vi "ProceListAction2.vi"(9 "Btn_AutoRun":refnum<vi>, 11 "AutoRunFlg":refnum<vi>) -> (0 "error out":errorcluster, 2 "pause":bool)   [LabVIEW 2019]
uses:
  Ctrl/MainPage UI Ref_VirbVision.ctl
  Function/Main UI/Glb/Main_UI Gb.vi
  LLB/Message/MsgShowAndLog.lvlib
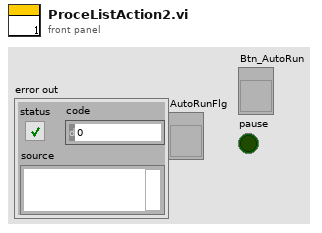
[diagram p1: front panel]
types:
  T1 = typedef "MainPage UI Ref_VirbVision.ctl" = cluster{"ProcessList":refnum<vi>, "Result Arr":refnum<vi>, "StopReceiveCmd":refnum<vi>}
  T2 = enum16{"Initial", "Write", "Read", "Save", "Load", "WrteAll"}
  T3 = enum16{"initial", "write", "add", "delete", "Load", "Save", "Read", "ReadProjectName"}
  T4 = cluster{"ProjectName":string, "Parameter":string[][]}[]
  T5 = cluster{"ProjectName":string, "Parameter":string[][]}
  T6 = cluster{"ROI":string, "Numbers":i32, "Data":string[][]}[]
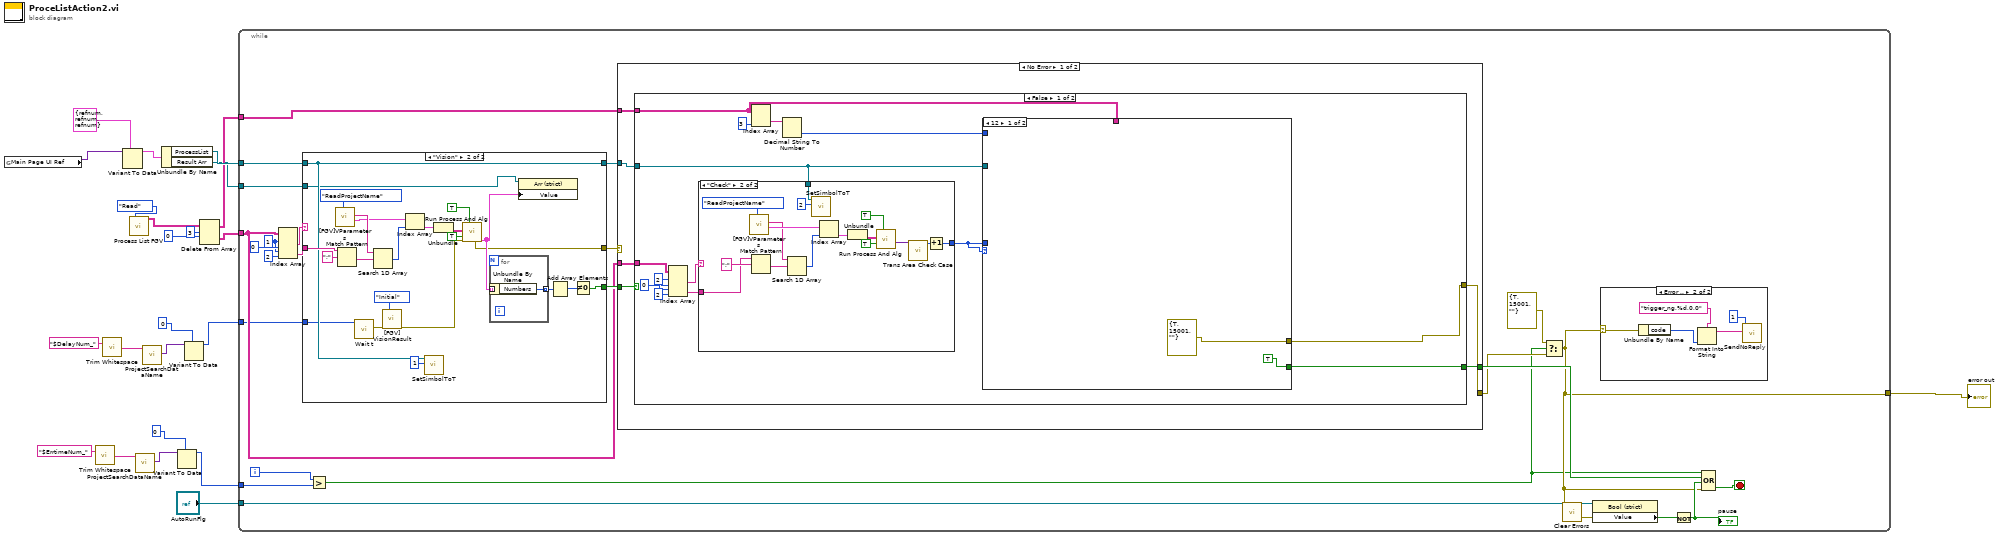
[diagram p0: block diagram]
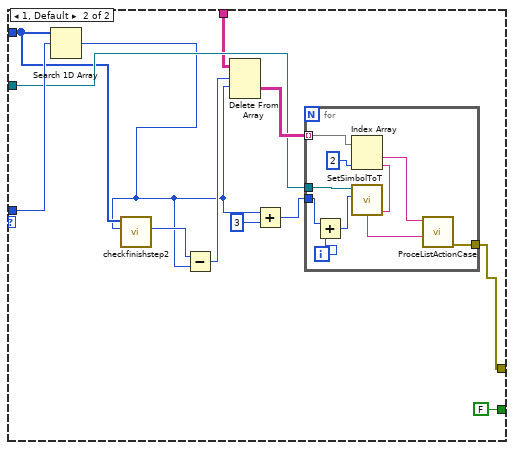
[diagram p2: hidden frame]
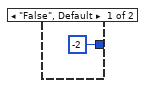
[diagram p3: hidden frame]
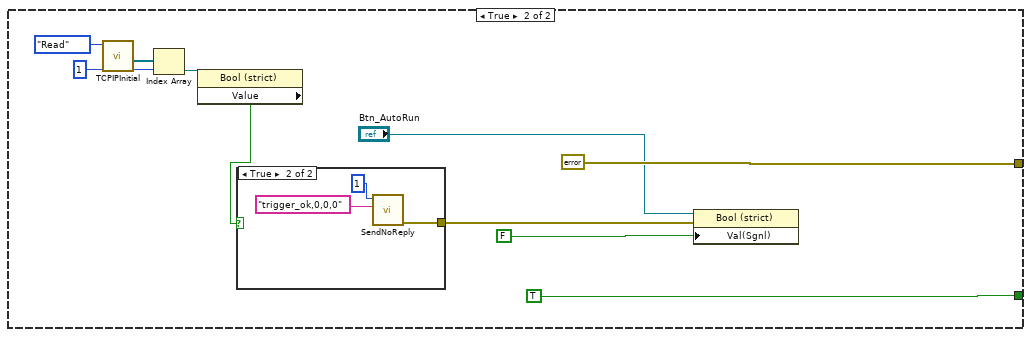
[diagram p4: hidden frame]
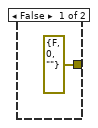
[diagram p5: hidden frame]
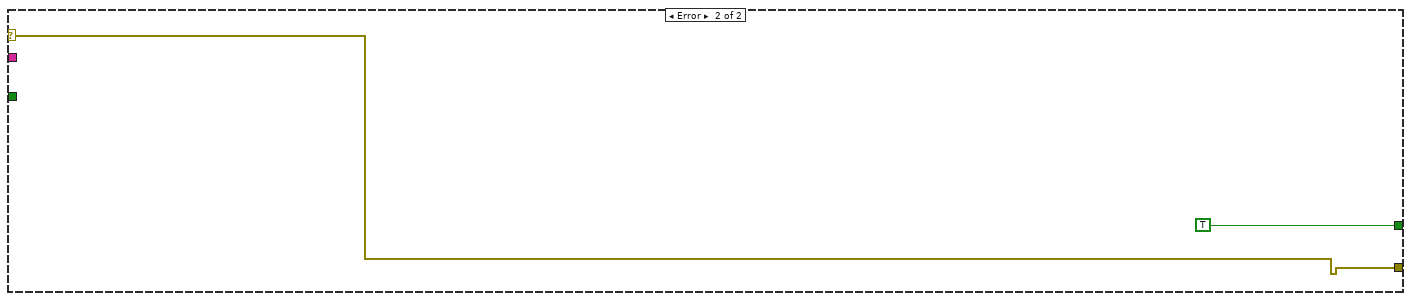
[diagram p6: hidden frame]
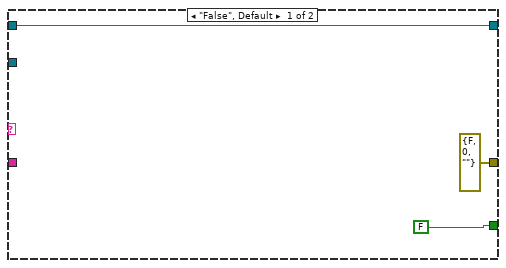
[diagram p7: hidden frame]
diagram:
  n1 = global read "Main_UI Gb.vi" "Main Page UI Ref"() -> (w2:variant)
  n2 = call <vilib>:"Trim Whitespace.vi"("string"="$ErrtimeNum_" ("element")) -> ("trimmed string"=w10:string)  [unwired: 1 in]
  n3 = call <vilib>:"Trim Whitespace.vi"("string"="$DelayNum_" ("element")) -> ("trimmed string"=w9:string)  [unwired: 1 in]
  n4 = Variant To Data(type=T1 {"ProcessList"=refnum, "Result Arr"=refnum, "StopReceiveCmd"=refnum} ("Main Page UIRef"), Variant=w2) -> (data=w4:T1)  [unwired: 1 in, 1 out]
  n5 = call "Process List FGV.vi"("Action"=T2."Read") -> ("TableOut"=w19:string[][])  [unwired: 12 in, 2 out]
  n6 = call "ProjectSearchDataName.vi"("element"=w10) -> ("variant"=w13:variant)  [unwired: 7 in, 3 out]
  n7 = call "ProjectSearchDataName.vi"("element"=w9) -> ("variant"=w8:variant)  [unwired: 7 in, 3 out]
  n8 = Unbundle By Name(w4) -> ("ProcessList"=w22:refnum<vi>, "Result Arr"=w1:refnum<vi>)
  n9 = Variant To Data(type=0, Variant=w13) -> (data=w11:i32)  [unwired: 1 in, 1 out]
  n10 = Variant To Data(type=0, Variant=w8) -> (data=w5:i32)  [unwired: 1 in, 1 out]
  n11 = Delete From Array(array=w19, length=3, index (row)=0) -> (deleted portion=w16:string[][], array with subset deleted=w15:string[][])  [unwired: 1 in]
  n12 = while {
    tunnel: [w28] -> w21
    tunnel: w22 -> [w46]
    tunnel: "AutoRunFlg" -> [w44]
    tunnel: w16 -> [w33]
    tunnel: w15 -> [w32]
    tunnel: w11 -> [w30]
    tunnel: w5 -> [w25]
    tunnel: w1 -> [w24]
    i -> [w31]
    stop <- w48 stop-if-true
    w36 = 1 ("index (row)")
    n13 = Index Array(array=w33, index (row) #1=w36, index (col) #1=0 ("disabled index (col)"), index (row) #2=w36, index (col) #2=2 ("disabled index (col)")) -> (element #1=w37:string, element #2=w34:string)
    n14 = case shown="\"Vision\"" w37 {
      tunnel: w34 -> [_ w150]
      tunnel: [FALSE ("VisionOK") w138] -> w41
      tunnel: [w126 w131] -> w40
      tunnel: w46 -> [w126 w131]
      tunnel: [errorcluster {"status"=FALSE, "code"=0, "source"=""} ("error out") w132] -> w39
      tunnel: w25 -> [_ w129]
      tunnel: w24 -> [_ w128]
      frame "False", Default {
      }
      frame "Vision" {
        n15 = call "[FGV]VParameters.vi"("Enum"=T3."ReadProjectName") -> ("Data"=w144:T4, "ProjectName"=w147:string[])  [unwired: 7 in, 2 out]
        n16 = Match Pattern(string=w150, regular expression=";") -> (after substring=w146:string)  [unwired: 1 in, 3 out]
        n17 = call "Wait t.vi"("wait(ms)"=w129) -> ("error out"=w134:errorcluster)  [unwired: 10 in]
        n18 = Search 1D Array(1D array=w147, element=w146) -> (index of element=w145:i32)  [unwired: 1 in]
        n19 = call "[FGV] VisionResult.vi"("Action"=T2."Initial", "error in"=w134) -> ("error out"=w139:errorcluster)  [unwired: 11 in, 2 out]
        n20 = Index Array(array=w144, index=w145) -> (element=w143:T5)
        n21 = call "SetSimbolToT.vi"("index"=1, "ProcessList"=w131) -> ()  [unwired: 10 in]
        n22 = Unbundle(w143) -> ("Parameter"=w142:string[][])  [unwired: 1 out]
        n23 = call "Run Process And Alg.vi"("Process"=TRUE, "error in (no error)"=w139, "CheckDist"=TRUE, "ROIList"=w142) -> ("Result Arr"=w137:T6, "error out"=w132:errorcluster)  [unwired: 3 in, 3 out]
        n24 = for {
          tunnel: w137 -> [w152] mode=indexing
          tunnel: [w151] -> w136 mode=indexing
          n25 = Unbundle By Name(w152) -> ("Numbers"=w151:i32)
        }
        n26 = property class="Arr (strict)"(reference=w128, "Value"=w137) -> ()  [unwired: 1 in, 2 out]
        n27 = Add Array Elements(numeric array=w136) -> (sum=w135:i32)
        n28 = Not Equal To 0?(x=w135) -> (x != 0?=w138:bool)
      }
    }
    n29 = Greater?(x=w31, y=w30) -> (0:w27:bool)
    n30 = case shown="No Error" w39 {
      selector: w39 -> [_ w123]
      tunnel: w41 -> [w54 _]
      tunnel: [w53 w123] -> w29
      tunnel: [w52 TRUE] -> w47
      tunnel: w40 -> [w51 _]
      tunnel: w33 -> [w50 _]
      tunnel: w32 -> [w49 _]
      frame No Error {
        n31 = case shown="False" w54 {
          tunnel: [w57 errorcluster {"status"=FALSE, "code"=0, "source"="視覺結束"} ("error out")] -> w53
          tunnel: [w56 TRUE] -> w52
          tunnel: w51 -> [w55 _]
          tunnel: w50 -> [w68 _]
          tunnel: w49 -> [w60 _]
          frame False {
            w67 = 2 ("index (row)")
            n32 = Index Array(array=w68, index (row) #1=w67, index (col) #1=0 ("disabled index (col)"), index (row) #2=w67, index (col) #2=2 ("disabled index (col)")) -> (element #1=w63:string, element #2=w64:string)
            n33 = case shown="\"Check\"" w63 {
              tunnel: w64 -> [_ w98]
              tunnel: [-2 w95] -> w58
              tunnel: w55 -> [_ w93]
              frame "False", Default {
              }
              frame "Check" {
                n34 = call "[FGV]VParameters.vi"("Enum"=T3."ReadProjectName") -> ("Data"=w104:T4, "ProjectName"=w101:string[])  [unwired: 7 in, 2 out]
                n35 = Match Pattern(string=w98, regular expression=";") -> (after substring=w102:string)  [unwired: 1 in, 3 out]
                n36 = Search 1D Array(1D array=w101, element=w102) -> (index of element=w103:i32)  [unwired: 1 in]
                n37 = call "SetSimbolToT.vi"("index"=2, "ProcessList"=w93) -> ()  [unwired: 10 in]
                n38 = Index Array(array=w104, index=w103) -> (element=w105:T5)
                n39 = Unbundle(w105) -> ("Parameter"=w106:string[][])  [unwired: 1 out]
                n40 = call "Run Process And Alg.vi"("Process"=TRUE, "CheckDist"=TRUE, "ROIList"=w106) -> ("DetectOut"=w97:variant[])  [unwired: 4 in, 4 out]
                n41 = call "Trans Area Check Case.vi"("ResultIn"=w97) -> ("Case"=w96:i32)  [unwired: 10 in]
                n42 = Increment(x=w96) -> (x+1=w95:i32)
              }
            }
            n43 = Index Array(array=w60, index (col)=3 ("disabled index (col)")) -> (element=w61:string[])  [unwired: 1 in]
            n44 = Decimal String To Number(string=w61) -> (number=w59:i32[])  [unwired: 2 in, 1 out]
            n45 = case shown="12" w58 {
              tunnel: w58 -> [_ w82]
              tunnel: w55 -> [_ w78]
              tunnel: w60 -> [_ w77]
              tunnel: w59 -> [_ w76]
              tunnel: [errorcluster {"status"=TRUE, "code"=15001, "source"=""} ("t") w75] -> w57
              tunnel: [TRUE FALSE] -> w56
              frame 12 {
              }
              frame 1, Default {
                n46 = Search 1D Array(1D array=w76, element=w82) -> (index of element=w72:i32)  [unwired: 1 in]
                n47 = call "checkfinishstep2.vi"("Index"=w72, "StepNumber"=w76) -> ("Index"=w81:i32)  [unwired: 7 in, 2 out]
                n48 = Subtract(x=w81, y=w72) -> (x-y=w79:i32)
                n49 = Delete From Array(array=w77, length=w79, index (row)=w72) -> (deleted portion=w80:string[][])  [unwired: 1 in, 1 out]
                n50 = Add(x=w72, y=3) -> (x+y=w73:i32)
                n51 = for {
                  tunnel: [w91] -> w75
                  tunnel: w80 -> [w90] mode=indexing
                  tunnel: w78 -> [w86]
                  tunnel: w73 -> [w83]
                  i -> [w85]
                  n52 = Add(x=w83, y=w85) -> (x+y=w84:i32)
                  n53 = Index Array(array=w90, index #2=2 ("index")) -> (element #1=w89:string, element #2=w88:string)  [unwired: 1 in]
                  n54 = call "SetSimbolToT.vi"("index"=w84, "ProcessList"=w86) -> ()  [unwired: 10 in]
                  n55 = call "ProceListActionCase.vi"("DataIn"=w88, "TypeIn"=w89) -> ("error out"=w91:errorcluster)  [unwired: 9 in]
                }
              }
            }
          }
          frame True {
            n56 = call "TCPIPInitial.vi"("Enum"=enum16{"initial", "Read", "release"}."Read") -> ("Connect"=w112:refnum<vi>[])  [unwired: 7 in, 3 out]
            n57 = Index Array(array=w112, index=1) -> (element=w110:refnum<vi>)
            n58 = property class="Bool (strict)"(reference=w110) -> ("Value"=w109:bool)  [unwired: 1 in, 2 out]
            n59 = case shown="True" w109 {
              tunnel: [errorcluster {"status"=FALSE, "code"=0, "source"=""} ("error out") w120] -> w115
              frame False {
              }
              frame True {
                n60 = call "SendNoReply.vi"("DataIn"="trigger_ok,0,0,0", "index"=1) -> ("error out"=w120:errorcluster)  [unwired: 9 in]
              }
            }
            n61 = property class="Bool (strict)"(reference="Btn_AutoRun", error in=w115, "Val(Sgnl)"=FALSE ("Value")) -> ()  [unwired: 2 out]
          }
        }
      }
      frame Error {
      }
    }
    n62 = Select(t=errorcluster {"status"=TRUE, "code"=15001, "source"=""}, s=w27, f=w29) -> (s? t:f=w28:errorcluster)
    n63 = call <vilib>:"Clear Errors.vi"("error in (no error)"=w28) -> ("error out"=w43:errorcluster)  [unwired: 5 in, 1 out]
    n64 = property class="Bool (strict)"(reference=w44, error in=w43) -> ("Value"=w45:bool)  [unwired: 2 out]
    n65 = case shown="Error .." w28 {
      selector: w28 -> [_ w156]
      frame No Error {
      }
      frame Error {
        n66 = Unbundle By Name(w156) -> ("code"=w154:i32)
        n67 = Format Into String(format string="trigger_ng,%d,0,0" ("DataIn"), w154) -> (resulting string=w153:string)  [unwired: 2 in, 1 out]
        n68 = call "SendNoReply.vi"("DataIn"=w153, "index"=1) -> ()  [unwired: 9 in, 1 out]
      }
    }
    n69 = Not(x=w45) -> (.not. x?=w42:bool)
    "pause" <- w42
    n70 = Compound Arithmetic op=OR(w27, w47, w42, w28) -> (w48:bool)
  }
  "error out" <- w21
